vi "Oven Pattern Tool.vi"() -> ()   [LabVIEW 2018, in "Configuration.lvlib"]
uses:
  Configuration.lvlib
  Configuration.lvclass
panel:
  in  "Available Patterns":u16(ring) items=["M7-60", "M7-80", "M11-25"]
  out "Pattern Time (m)":string
  out "Pattern Temp":string
  out "Active Pattern":string
  in  "Update Pattern":bool
  in  "stop":bool
  in  "Device":string="Oven"
  in  "Select Device":bool
  in  "Read pattern":bool
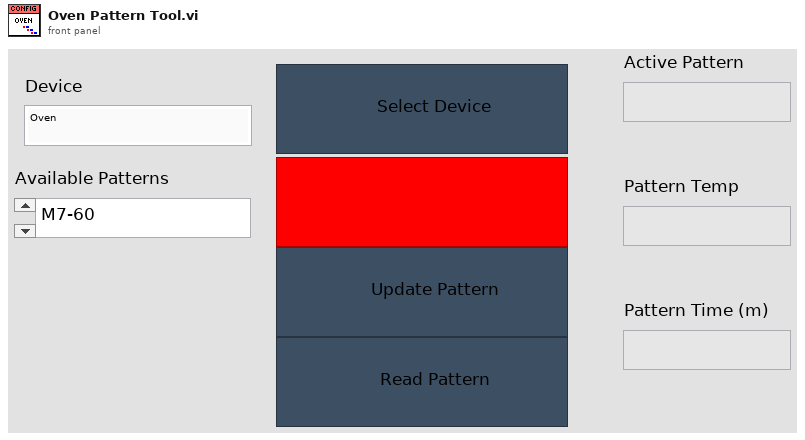
[diagram p1: front panel]
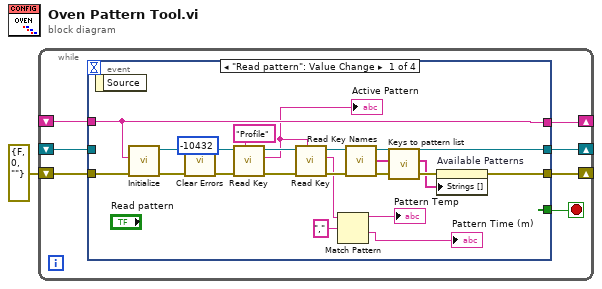
[diagram p0: block diagram]
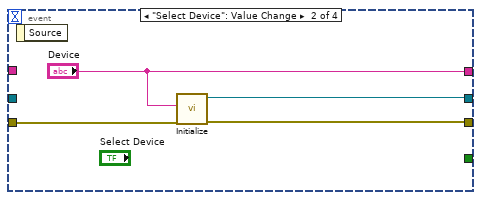
[diagram p2: hidden frame]
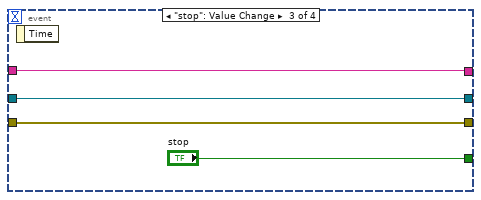
[diagram p3: hidden frame]
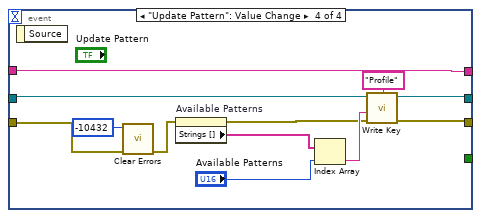
[diagram p4: hidden frame]
diagram:
  n1 = while {
    shift-right: [w6] -> _
    shift-left: errorcluster {"status"=FALSE, "code"=0, "source"=""} ("error out") -> [w7]
    shift-right: [w4] -> _
    shift-left: _ -> [w5]
    shift-right: [w2] -> _
    shift-left: _ -> [w3]
    stop <- w8 stop-if-true
    n2 = event shown="[0] \"Read pattern\": Value Change" {
      selector: _ -> [_ _ _ _]
      dyn-events: _ -> [_ _ _ _]
      timeout: _ -> [_ _ _ _]
      tunnel: [_ _ "stop" _] -> w8
      tunnel: w7 -> [w28 w33 w36 w45]
      tunnel: [w20 w30 w36 w49] -> w6
      tunnel: w5 -> [_ _ w35 w47]
      tunnel: [w22 w32 w35 w48] -> w4
      tunnel: w3 -> [w26 _ w34 w46]
      tunnel: [w26 "Device" w34 w46] -> w2
      event "Read pattern": Value Change {
        n3 = event-data() -> ()  [unwired: 1 in, 1 out]
        n4 = call "Initialize.vi"("error in"=w28, "Device"=w26) -> ("error out"=w27:errorcluster, "Configuration out"=w25:refnum<class "Configuration.lvclass">)  [unwired: 8 in]
        n5 = call <vilib>:"Clear Errors.vi"("error in (no error)"=w27, "specific error code to clear (0: all)"=-10432) -> ("error out"=w24:errorcluster)  [unwired: 4 in, 1 out]
        n6 = call "Read Key.vi"("Key:"="Profile", "error in"=w24, "Configuration in"=w25) -> ("error out"=w19:errorcluster, "Value"=w17:string, "Configuration out"=w18:refnum<class "Configuration.lvclass">)  [unwired: 6 in]
        "Active Pattern" <- w17
        n7 = call "Read Key.vi"("Key:"=w17, "error in"=w19, "Configuration in"=w18) -> ("error out"=w15:errorcluster, "Value"=w14:string, "Configuration out"=w16:refnum<class "Configuration.lvclass">)  [unwired: 6 in]
        n8 = Match Pattern(string=w14, regular expression=",") -> (before substring=→"Pattern Temp":string, after substring=→"Pattern Time (m)":string)  [unwired: 1 in, 2 out]
        n9 = call "Read Key Names.vi"("error in"=w15, "Configuration in"=w16) -> ("error out"=w21:errorcluster, "Keys"=w10:string[], "Configuration out"=w22:refnum<class "Configuration.lvclass">)  [unwired: 7 in]
        n10 = call "Keys to pattern list.vi"("Keys"=w10) -> ("Pattern List"=w9:string[])  [unwired: 10 in]
        n11 = property on="Available Patterns" class="Ring (strict)"(error in=w21, "Strings []"=w9) -> (error out=w20:errorcluster)  [unwired: 1 in, 1 out]
      }
      event "Select Device": Value Change {
        n12 = event-data() -> ()  [unwired: 1 in, 1 out]
        n13 = call "Initialize.vi"("error in"=w33, "Device"="Device") -> ("error out"=w30:errorcluster, "Configuration out"=w32:refnum<class "Configuration.lvclass">)  [unwired: 8 in]
      }
      event "stop": Value Change {
        n14 = event-data() -> ()  [unwired: 1 in, 1 out]
      }
      event "Update Pattern": Value Change {
        n15 = event-data() -> ()  [unwired: 1 in, 1 out]
        n16 = call <vilib>:"Clear Errors.vi"("error in (no error)"=w45, "specific error code to clear (0: all)"=-10432) -> ("error out"=w39:errorcluster)  [unwired: 4 in, 1 out]
        n17 = property on="Available Patterns" class="Ring (strict)"(error in=w39) -> (error out=w38:errorcluster, "Strings []"=w41:string[])  [unwired: 1 in, 1 out]
        n18 = Index Array(array=w41, index="Available Patterns") -> (element=w40:string)
        n19 = call "Write Key.vi"("error in"=w38, "value"=w40, "key"="Profile", "Configuration in"=w47) -> ("error out"=w49:errorcluster, "Configuration out"=w48:refnum<class "Configuration.lvclass">)  [unwired: 6 in]
      }
    }
  }
